vi "Open.vi"(8 "error in (no error)":errorcluster, 11 "File in":refnum<class "File.lvclass">) -> (0 "error out":errorcluster, 3 "File out":refnum<class "File.lvclass">)   [LabVIEW 2020, in "File.lvclass"]
uses:
  File.lvclass
  File.lvclass/File.ctl
  Read Data File  Path.vi
  Read Is open.vi
  Read tdms stream.vi
  Write tdms stream.vi
  Write Is open.vi
  Metadata/Metadata.lvclass
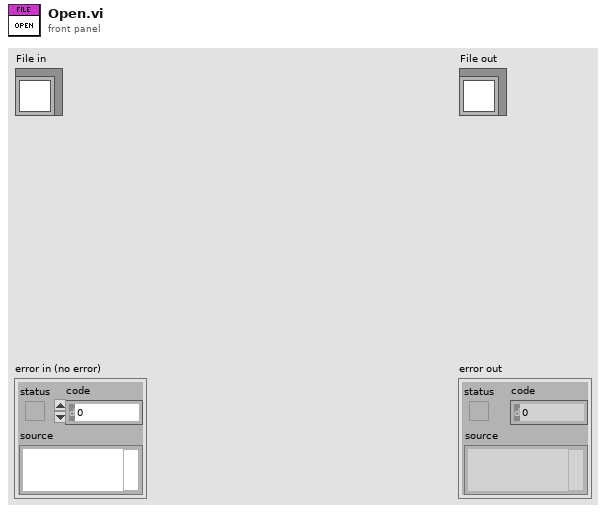
[diagram p1: front panel]
types:
  T1 = enum16{"open", "open or create", "create or replace", "create", "open (read-only)"}
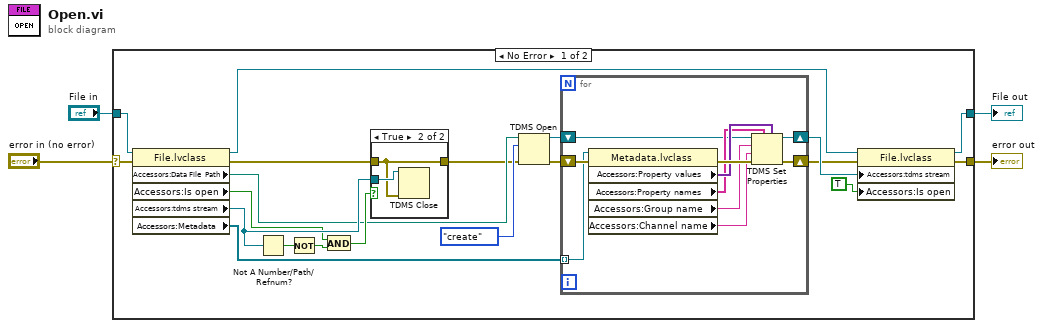
[diagram p0: block diagram]
diagram:
  n1 = case shown="No Error" "error in (no error)" {
    selector: "error in (no error)" -> [w24 w39]
    tunnel: [w15 w39] -> w3
    tunnel: [w13 w38] -> w1
    tunnel: "File in" -> [w23 w38]
    frame No Error {
      n2 = property class="File.lvclass"(reference=w23, error in=w24) -> (reference out=w14:refnum<class "File.lvclass">, error out=w11:errorcluster, "Accessors:Data File  Path"=w17:path, "Accessors:Is open"=w18:bool, "Accessors:tdms stream"=w20:refnum<k34>, "Accessors:Metadata"=w9:refnum<class "Metadata.lvclass">[])
      n3 = Not A Number/Path/Refnum?(number/path/refnum=w20) -> (NaN/Path/Refnum?=w21:bool)
      n4 = Not(x=w21) -> (.not. x?=w22:bool)
      n5 = And(x=w18, y=w22) -> (x .and. y?=w19:bool)
      n6 = case shown="True" w19 {
        tunnel: w11 -> [w35 w36]
        tunnel: w20 -> [_ w37]
        tunnel: [w35 w36] -> w10
        frame False {
        }
        frame True {
          n7 = TDMS Close(8:w36, 11:w37) -> ()  [unwired: 2 out]
        }
      }
      n8 = TDMS Open(8:w10, 10:T1."create" ("operation (0:open)"), 11:w17) -> (0:w6:errorcluster, 3:w8:refnum<k34>)  [unwired: 4 in]
      n9 = for {
        tunnel: w9 -> [w30] mode=indexing
        shift-right: [w34] -> w7
        shift-left: w8 -> [w25]
        shift-right: [w33] -> w5
        shift-left: w6 -> [w32]
        n10 = property class="Metadata.lvclass"(reference=w30, error in=w32) -> (error out=w31:errorcluster, "Accessors:Property values"=w29:variant[], "Accessors:Property names"=w28:string[], "Accessors:Group name"=w27:string, "Accessors:Channel name"=w26:string)  [unwired: 1 out]
        n11 = TDMS Set Properties(5:w29, 7:w28, 8:w31, 9:w26, 10:w27, 11:w25) -> (0:w33:errorcluster, 3:w34:refnum<k34>)  [unwired: 2 out]
      }
      n12 = property class="File.lvclass"(reference=w14, error in=w5, "Accessors:tdms stream"=w7, "Accessors:Is open"=TRUE ("Is open")) -> (reference out=w13:refnum<class "File.lvclass">, error out=w15:errorcluster)
    }
    frame Error {
    }
  }
  "error out" <- w3
  "File out" <- w1
